vi "LabViewTCPClient.vi"() -> ()   [LabVIEW 2016]
uses:
  <vilib>/Platform/TimedLoop/XDataNode/timing_clust.ctl
  <vilib>/Platform/TimedLoop/XDataNode/nitl_modes.ctl
  <vilib>/Platform/TimedLoop/XDataNode/wakeup.ctl
  <vilib>/Platform/TimedLoop/XDataNode/XDataNode.xnode
  <vilib>/Platform/TimedLoop/XDataNode/XDNodeRunTimeDep.lvlib
panel:
  out "Error Loop Counter 2":dbl
  in  "Error Loop Counter":dbl
  in  "LabView Client ID":string="PI3_TCP_LV_Client"
  out "decimal integer string":string="2"
  out "bytes written":i32=1
  in  "HEADER":dbl=64.0
  in  "Dt":dbl=5000.0
  in  "HeartBeat":dbl
  in  "Stop LabView Client":bool
  in  "IP":string="localhost"
  in  "PORT":dbl=5506.0
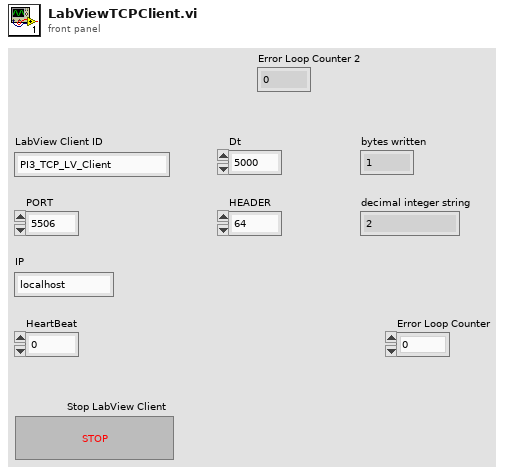
[diagram p1: front panel]
types:
  T1 = typedef "XDNodeRunTimeDep.lvlib/timing_clust.ctl" = cluster{"Expected End [f-1]":u64, "Actual End [f-1]":u64, "Finished Late? [f-1]":bool, "Expected End [i-1]":u64, "Actual End [i-1]":u64, "Finished Late? [i-1]":bool, "Expected Start [i]":u64, "Actual Start [i]":u64, "Expected Start [f]":u64, "Actual Start [f]":u64, "Source Name":string, "Structure Name":string, "Period":i64, "Deadline":i64, "Offset":i64, "Start":i64, "Priority":i32, "Timeout":i32, "Mode":T2, "Wakeup Reason":T3, "Error":errorcluster, "Source Type":string, "Secondary Source Type":string, "Global End Time":u64, "Global Start Time":u64, "Frame Duration":u64, "Iteration Duration":u64, "Assigned CPU":i32, "I/O Scan Engine Mode":u32}
  T2 = typedef "XDNodeRunTimeDep.lvlib/nitl_modes.ctl" = enum32{"No Change", "Process missed periods, maintain original phase", "Discard missed periods, maintain original phase", "Process missed periods, ignore original phase", "Discard missed periods, ignore original phase"}
  T3 = typedef "XDNodeRunTimeDep.lvlib/wakeup.ctl" = enum32{"Normal", "Aborted", "Asynchronous wakeup", "Timing source error", "Timed loop error", "Timeout"}
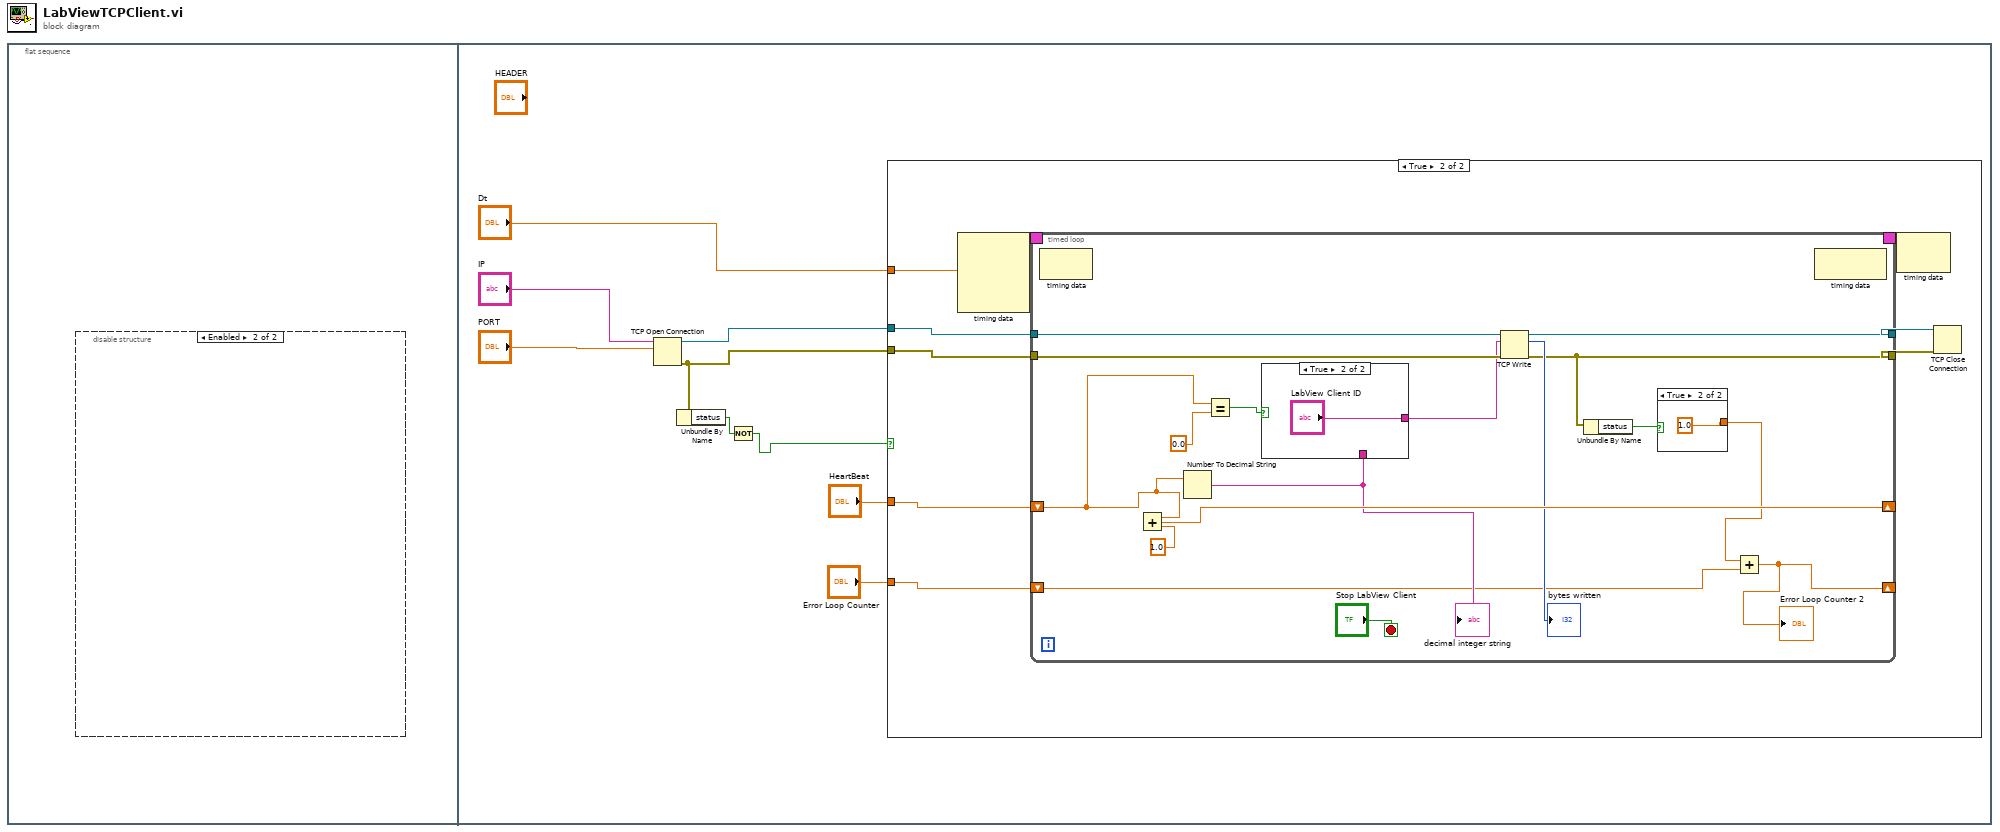
[diagram p0: block diagram]
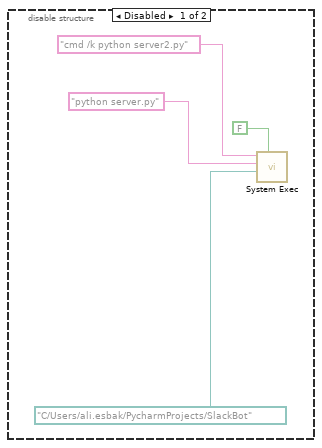
[diagram p2: hidden frame]
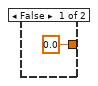
[diagram p4: hidden frame]
diagram:
  n1 = flat-sequence {
    frame #0 {
      n2 = disable-structure shown="Enabled" {
        frame Disabled {
          n3 = call <vilib>:"System Exec.vi"("wait until completion? (T)"=FALSE, "working directory"=path "C:/Users/ali.esbak/PycharmProjects/SlackBot", "standard input"="python server.py", "command line"="cmd /k python server2.py") -> ()  [unwired: 4 in, 4 out]
        }
        frame Enabled {
        }
      }
    }
    frame #1 {
      n4 = TCP Open Connection(address="IP", remote port or service name="PORT") -> (connection ID=w11:refnum<k5>, error out=w7:errorcluster)  [unwired: 3 in]
      n5 = Unbundle By Name(w7) -> ("status"=w6:bool)
      n6 = Not(x=w6) -> (.not. x?=w5:bool)
      n7 = case shown="True" w5 {
        tunnel: "HeartBeat" -> [_ w20]
        tunnel: "Dt" -> [_ w19]
        tunnel: w7 -> [_ w16]
        tunnel: w11 -> [_ w15]
        tunnel: "Error Loop Counter" -> [_ w14]
        frame False {
          # "we have a tcp error try to reconnect"
        }
        frame True {
          n8 = node-c288(w19) -> (w22:T1)  [unwired: 3 in]
          n9 = timed-loop {
            timing: w22 -> [_]
            timing-out: [_] -> w21
            tunnel: w15 -> [w39]
            tunnel: w16 -> [w38]
            tunnel: [w37] -> w17
            tunnel: [w27] -> w18
            shift-right: [w34] -> _
            shift-left: w20 -> [w32]
            shift-right: [w23] -> _
            shift-left: w14 -> [w25]
            stop <- "Stop LabView Client" stop-if-true
            n10 = node-c288() -> ()  [unwired: 1 in, 1 out]
            n11 = Add(x=w32, y=1.0) -> (x+y=w34:dbl)
            n12 = Number To Decimal String(number=w32) -> (decimal integer string=w28:string)  [unwired: 1 in]
            "decimal integer string" <- w28
            n13 = Equal?(x=w32, y=0.0) -> (x = y?=w30:bool)
            n14 = case shown="True" w30 {
              tunnel: [w42 "LabView Client ID"] -> w29
              tunnel: w28 -> [w42 _]
              frame False {
              }
              frame True {
              }
            }
            n15 = TCP Write(connection ID=w39, data in=w29, error in (no error)=w38) -> (connection ID out=w37:refnum<k5>, bytes written=→"bytes written":i32, error out=w27:errorcluster)  [unwired: 1 in]
            n16 = Unbundle By Name(w27) -> ("status"=w26:bool)
            n17 = case shown="True" w26 {
              tunnel: [0.0 ("Error Loop Counter") 1.0 ("Error Loop Counter")] -> w24
              frame False {
              }
              frame True {
              }
            }
            n18 = Add(x=w24, y=w25) -> (x+y=w23:dbl)
            "Error Loop Counter 2" <- w23
            n19 = node-c288() -> ()  [unwired: 1 in, 1 out]
          }
          n20 = node-c288(w21) -> ()  [unwired: 1 out]
          n21 = TCP Close Connection(connection ID=w17, error in (no error)=w18) -> ()  [unwired: 1 in, 2 out]
        }
      }
    }
  }
